vi "PDE_SpMtrx_CG Solver.vi"(6 "termination":cluster{"max iter":i32, "tolerance":dbl}={"max iter"=200, "tolerance"=1e-08}, 8 "error in (no error)":errorcluster, 9 "X0":dbl[](array[numeric]), 10 "RHS":dbl[](array[numeric]), 11 "Sparse Mtrx":T1) -> (0 "error out":errorcluster, 3 "X":dbl[](array[numeric]))   [LabVIEW 2020, in "NI_PDE.lvlib"]
uses:
  <vilib>/gmath/NI_PDE.lvlib
  <vilib>/gmath/pde.llb/Common/PDE_Sparse Mtrx.ctl
  <vilib>/Analysis/baseanly.llb/Real Dot Product.vi
  <vilib>/Analysis/NI_AALBase.lvlib
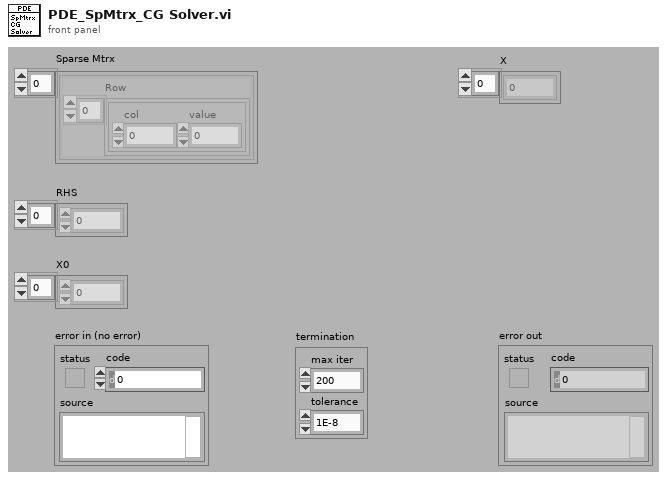
[diagram p1: front panel]
types:
  T1 = typedef "NI_PDE.lvlib/PDE_Sparse Mtrx.ctl" = cluster{"Row":cluster{"col":i32, "value":dbl}[]}[]
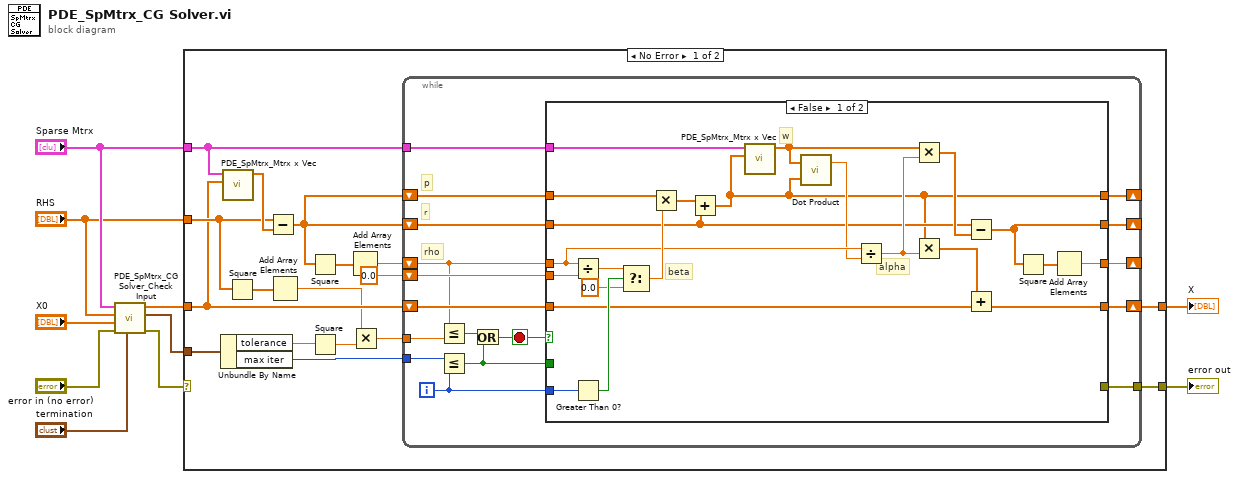
[diagram p0: block diagram]
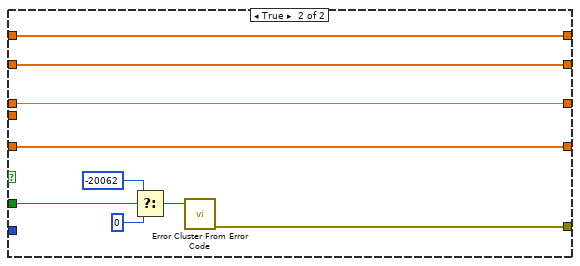
[diagram p2: hidden frame]
diagram:
  n1 = call <vilib>:"PDE_SpMtrx_CG Solver_Check Input.vi"("termination in"="termination", "error in (no error)"="error in (no error)", "X0 In"="X0", "RHS"="RHS", "Sparse Mtrx"="Sparse Mtrx") -> ("error out"=w2:errorcluster, "termination out"=w4:cluster{"max iter":i32, "tolerance":dbl}, "X0 Out"=w3:dbl[])  [unwired: 4 out]
  n2 = case shown="No Error" w2 {
    selector: w2 -> [_ w76]
    tunnel: w4 -> [w26 _]
    tunnel: w3 -> [w12 _]
    tunnel: "Sparse Mtrx" -> [w22 _]
    tunnel: "RHS" -> [w15 _]
    tunnel: [w21 _] -> w10
    tunnel: [w13 w76] -> w9
    frame No Error {
      n3 = Unbundle By Name(w26) -> ("tolerance"=w24:dbl, "max iter"=w25:i32)
      n4 = call <vilib>:"PDE_SpMtrx_Mtrx x Vec.vi"("X"=w12, "Sparse Mtrx"=w22) -> ("Mtrx x X"=w27:dbl[])  [unwired: 9 out]
      n5 = Square(x=w15) -> (x^2=w16:dbl[])
      n6 = Subtract(x=w15, y=w27) -> (x-y=w17:dbl[])
      n7 = Add Array Elements(numeric array=w16) -> (sum=w11:dbl)
      n8 = Square(x=w17) -> (x^2=w20:dbl[])
      n9 = Square(x=w24) -> (x^2=w14:dbl)
      n10 = Add Array Elements(numeric array=w20) -> (sum=w19:dbl)
      n11 = Multiply(x=w11, y=w14) -> (x*y=w23:dbl)
      n12 = while {
        tunnel: w23 -> [w44]
        shift-right: [w40] -> w21
        shift-left: w12 -> [w41]
        shift-right: [w33] -> _
        shift-left: w17 -> [w37]
        tunnel: w25 -> [w43]
        tunnel: w22 -> [w34]
        shift-right: [w32] -> _
        shift-left: w19 -> [w31]
        shift-left: 0.0 ("Numeric") -> [w38]
        shift-right: [w35] -> _
        shift-left: w17 -> [w36]
        tunnel: [w28] -> w13
        i -> [w39]
        stop <- w30 stop-if-true
        # "p"
        # "r"
        # "rho"
        n13 = Less Or Equal?(x=w31, y=w44) -> (x <= y?=w42:bool)
        n14 = Less Or Equal?(x=w43, y=w39) -> (x <= y?=w29:bool)
        n15 = Or(x=w42, y=w29) -> (x .or. y?=w30:bool)
        n16 = case shown="False" w30 {
          tunnel: w41 -> [w57 w74]
          tunnel: [w56 w74] -> w40
          tunnel: w39 -> [w66 _]
          tunnel: w31 -> [w59 w72]
          tunnel: w38 -> [w64 _]
          tunnel: w37 -> [w46 w73]
          tunnel: w36 -> [w48 w75]
          tunnel: [w45 w75] -> w35
          tunnel: w34 -> [w60 _]
          tunnel: [w50 w73] -> w33
          tunnel: [w49 w72] -> w32
          tunnel: w29 -> [_ w71]
          tunnel: [_ w67] -> w28
          frame False {
            # "alpha"
            # "w"
            # "beta"
            n17 = Divide(x=w59, y=w64) -> (x/y=w63:dbl)
            n18 = Greater Than 0?(x=w66) -> (x > 0?=w65:bool)
            n19 = Select(t=w63, s=w65, f=0.0) -> (s? t:f=w61:dbl)
            n20 = Multiply(x=w48, y=w61) -> (x*y=w47:dbl[])
            n21 = Add(x=w47, y=w46) -> (x+y=w45:dbl[])
            n22 = call <vilib>:"PDE_SpMtrx_Mtrx x Vec.vi"("X"=w45, "Sparse Mtrx"=w60) -> ("Mtrx x X"=w54:dbl[])  [unwired: 9 out]
            n23 = call-poly <vilib>:"Dot Product.vi"("Y Vector"=w45, "X Vector"=w54) -> ("X * Y"=w58:dbl)  [unwired: 1 out]
            n24 = Divide(x=w59, y=w58) -> (x/y=w53:dbl)
            n25 = Multiply(x=w54, y=w53) -> (x*y=w52:dbl[])
            n26 = Multiply(x=w45, y=w53) -> (x*y=w55:dbl[])
            n27 = Subtract(x=w46, y=w52) -> (x-y=w50:dbl[])
            n28 = Add(x=w55, y=w57) -> (x+y=w56:dbl[])
            n29 = Square(x=w50) -> (x^2=w51:dbl[])
            n30 = Add Array Elements(numeric array=w51) -> (sum=w49:dbl)
          }
          frame True {
            n31 = Select(t=-20062, s=w71, f=0) -> (s? t:f=w68:i32)
            n32 = call <vilib>:"Error Cluster From Error Code.vi"("error code (0)"=w68) -> ("error out"=w67:errorcluster)  [unwired: 2 in, 6 out]
          }
        }
      }
    }
    frame Error {
    }
  }
  "X" <- w10
  "error out" <- w9
